vi "Teleop-System-Acquire-Decide.vi"   [LabVIEW 2019]
uses:
  <vilib>/Rock Robotics/WPI/Joystick/WPI_JoystickArcadeMapping.vi
  Teleop-System-Globals.vi
types:
  T1 = typedef "WPI_JoystickDevRef.ctl" = cluster{"Device":T2}
  T2 = typedef "WPI_JoystickDeviceEnum.ctl" = enum16{"USB 0", "USB 1", "USB 2", "USB 3", "USB 4", "USB 5"}
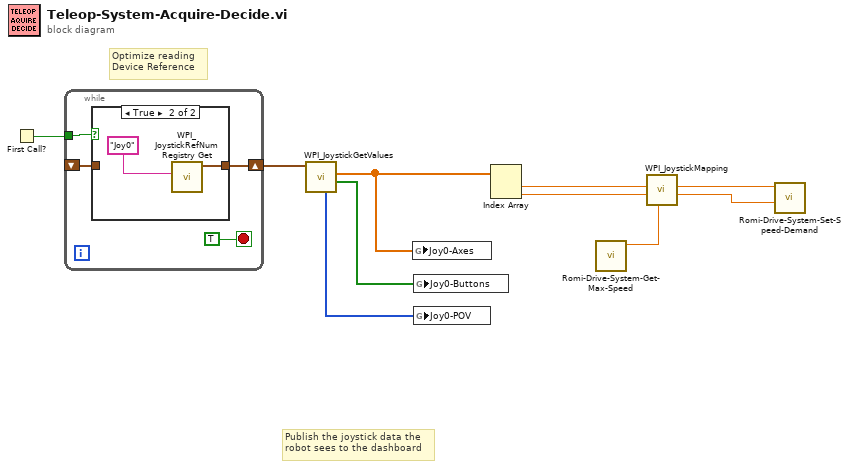
[diagram p0: block diagram]
diagram:
  # "Optimize reading \nDevice Reference"
  # "Publish the joystick data the\nrobot sees to the dashboard"
  n1 = First Call?() -> (First Call?: T/F=w5:bool)
  n2 = while {
    tunnel: w5 -> [w12]
    shift-right: [w14] -> w6
    shift-left: _ -> [w11]
    stop <- TRUE stop-if-true
    n3 = case shown="True" w12 {
      tunnel: [w15 w17] -> w14
      tunnel: w11 -> [w15 _]
      frame False {
      }
      frame True {
        n4 = call <vilib>:"WPI_JoystickRefNum Registry Get.vi"("refnum name"="Joy0") -> ("JoystickDevRef"=w17:T1)  [unwired: 1 in, 9 out]
      }
    }
  }
  n5 = call <vilib>:"WPI_JoystickGetValues.vi"("JoystickDevRef"=w6) -> ("Buttons"=w2:bool[], "Axes"=w3:dbl[], "POVs"=w1:i16[])  [unwired: 6 in, 2 out]
  n6 = global write "Teleop-System-Globals.vi" "Joy0-Axes"(w3) -> ()
  n7 = global write "Teleop-System-Globals.vi" "Joy0-Buttons"(w2) -> ()
  n8 = global write "Teleop-System-Globals.vi" "Joy0-POV"(w1) -> ()
  n9 = Index Array(array=w3) -> (element #1=w7:dbl, element #2=w8:dbl)  [unwired: 2 in]
  n10 = call "Romi-Drive-System-Get-Max-Speed.vi"() -> ("MaxSpeed-Ft/Sec"=w4:dbl)  [unwired: 11 in]
  n11 = call-poly <vilib>:"WPI_JoystickMapping.vi"("Max Output"=w4, "Y axis value"=w8, "X axis value"=w7) -> ("Right Motor Value"=w10:dbl, "Left Motor Value"=w9:dbl)  [unwired: 7 in]
  n12 = call "Romi-Drive-System-Set-Speed-Demand.vi"("Right Speed Demand"=w10, "Left Speed Demand"=w9) -> ()  [unwired: 10 in]
